vi "Create.vi"(7 "Direction":T1, 8 "error in (no error)":errorcluster, 9 "Custom Config Data":u8[](array[numeric]), 10 "Name":string, 11 "CIFTag in":refnum<class "CIFTagI64.lvclass">) -> (0 "error out":errorcluster, 3 "CIFTag out":refnum<class "CIFTagI64.lvclass">)   [LabVIEW 2021, in "CIFTagI64.lvclass"]
uses:
  CIFTagI64.lvclass
  D:/dev/CIF-LVCore/src/CIFUtilities/CIFChannels/CIFChannels.lvclass
  D:/dev/CIF-LVCore/src/Channels/CIFTag/CIFTag/CIFTag.lvclass
  CIFUtilities/CIFChannels/CIFChannels.lvclass/CIFChannels.ctl
  CIFTagI64.lvclass/CIFTagI64.ctl
  CIFTag/CIFTag.lvclass/CIFTag.ctl
  CIFUtilities/CIFChannels/Accessors/Write Channel State.vi
  CIFTag/Accessors/Write CIF Channel.vi
  CIFUtilities/CIFChannels/Accessors/Write Channel Class.vi
  CIFUtilities/CIFChannels/Accessors/Write Direction.vi
  CIFUtilities/CIFChannels/Accessors/Write Disconnect Behavior.vi
  CIFUtilities/CIFChannels/Accessors/Write Name.vi
  CIFUtilities/CIFChannels/Accessors/Write Custom Config Data.vi
  <vilib>/CIFChannels/SubVIs/Add Error.vi
  Create Publisher.vi/5c81bccc-e622-4fe9-9720-12299560a745.vi/c28b0ead-42ad-4072-80a2-aca7f2bd7ce3.vi
  <vilib>/CIFChannels/SubVIs/CIFServices Fill In Error Info Ex.vi
  <vilib>/CIFChannels/SubVIs/Get dll Path.vi
  Create Publisher.vi/522c0ff3-de7b-4614-b37e-c276d07c7241.vi/4bc1c15b-36ab-481f-b8dd-c64075ce723a.vi
  Create Publisher.vi/522c0ff3-de7b-4614-b37e-c276d07c7241.vi/d83cb72b-7713-41fc-a3d1-682de79cf574.vi
  <vilib>/CIFChannels/SubVIs/Append Error Location.vi
  CIFUtilities/CIFChannels/Typedef/Disconnect Behavior.ctl
  CIFUtilities/CIFChannels/CIFChannels.lvclass
  CIFUtilities/CIFChannels/Typedef/Channel State.ctl
  02edcf3a-6131-4746-b933-e6a1af1fcb43.vi
  62a89f15-4a42-416c-81d4-6d85d5f7b5c9.vi
  85493118-15d5-4bf2-af7e-e73f555693b8.vi
  4a91887f-a40d-4172-85c4-b368c6e6f55f.vi
  D:/dev/CIF-LVCore/src/Channels/CIFTag/I64/CIFTagI64.lvclass
  CIFUtilities/CIFChannels/Typedef/Direction.ctl
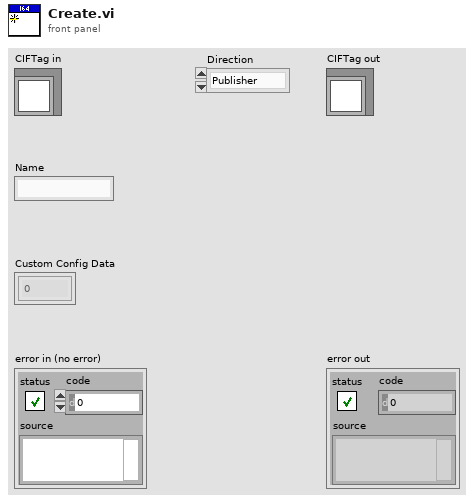
[diagram p1: front panel]
types:
  T1 = typedef "CIFChannels.lvclass/Direction.ctl" = enum16{"Publisher", "Subscriber"}
  T2 = typedef "CIFChannels.lvclass/Disconnect Behavior.ctl" = enum16{"Default value", "Last value", "Error with default"}
  T3 = typedef "CIFChannels.lvclass/Channel State.ctl" = enum16{"Creating", "Disconnected", "Connecting", "Connected", "Destroying"}
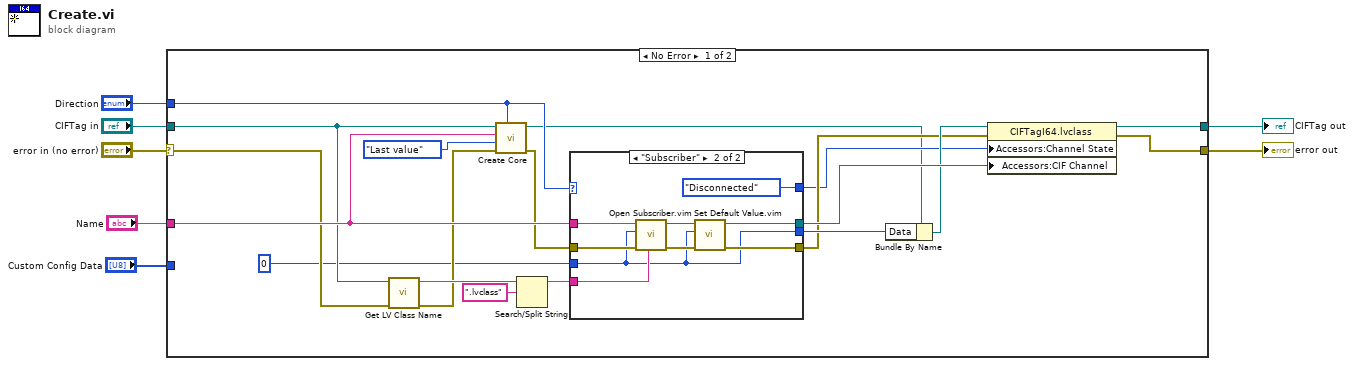
[diagram p0: block diagram]
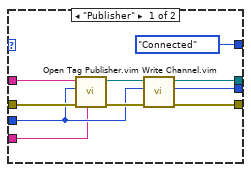
[diagram p2: hidden frame]
diagram:
  n1 = case shown="No Error" "error in (no error)" {
    selector: "error in (no error)" -> [w13 w47]
    tunnel: [w25 w47] -> w5
    tunnel: [w18 w46] -> w6
    tunnel: "CIFTag in" -> [w17 w46]
    tunnel: "Name" -> [w24 _]
    tunnel: "Direction" -> [w11 _]
    tunnel: "Custom Config Data" -> [_ _]
    frame No Error {
      n2 = call <vilib>:"Get LV Class Name.vi"("error in (no error)"=w13, "object"=w17) -> ("error out"=w12:errorcluster, "class name"=w16:string)  [unwired: 8 in]
      n3 = call "Create Core.vi"("Direction"=w11, "error in (no error)"=w12, "Disconnect Behavior"=Disconnect_Behavior."Last value", "Name"=w24, "CIFChannels in"=w17) -> ("error out"=w23:errorcluster, "CIFChannels out"=w9:refnum<class "CIFTagI64.lvclass">)  [unwired: 5 in]
      n4 = Search/Split String(string=w16, search string/char (-)=".lvclass") -> (substring before match=w14:string)  [unwired: 1 in, 2 out]
      n5 = case shown="\"Subscriber\"" w11 {
        tunnel: w24 -> [w36 w44]
        tunnel: w23 -> [w35 w43]
        tunnel: [w32 w40] -> w22
        tunnel: i64 0 ("Default Value") -> [w31 w37]
        tunnel: [w30 w37] -> w20
        tunnel: [w29 w39] -> w19
        tunnel: w14 -> [w28 w38]
        tunnel: [Channel_State."Connected" ("Channel State") Channel_State."Disconnected" ("Channel State")] -> w10
        frame "Publisher" {
          n6 = call "Open Tag Publisher.vim"("Channel Type Description"=w28, "error in"=w35, "Input Type"=w31, "Channel Name"=w36) -> ("error out"=w33:errorcluster, "CIF Channel"=w34:refnum<k21>)  [unwired: 6 in]
          n7 = call "Write Channel.vim"("error in"=w33, "Data in"=w31, "CIF Channel in"=w34) -> ("error out"=w29:errorcluster, "Data out"=w30:i64, "CIF Channel out"=w32:refnum<k21>)  [unwired: 5 in, 1 out]
        }
        frame "Subscriber" {
          n8 = call "Open Subscriber.vim"("Channel Type Description"=w38, "error in"=w43, "Input Type"=w37, "Channel Name"=w44) -> ("error out"=w42:errorcluster, "CIF Channel"=w41:refnum<k21>)  [unwired: 6 in]
          n9 = call "Set Default Value.vim"("error in"=w42, "Data in"=w37, "CIF Channel in"=w41) -> ("error out"=w39:errorcluster, "CIF Channel out"=w40:refnum<k21>)  [unwired: 7 in]
        }
      }
      n10 = Bundle By Name(cluster=w9, "Data"=w20) -> (w21:refnum<class "CIFTagI64.lvclass">)
      n11 = property class="CIFTagI64.lvclass"(reference=w21, error in=w19, "Accessors:Channel State"=w10, "Accessors:CIF Channel"=w22) -> (reference out=w18:refnum<class "CIFTagI64.lvclass">, error out=w25:errorcluster)
    }
    frame Error {
    }
  }
  "error out" <- w5
  "CIFTag out" <- w6
